vi "Calculate 1 digit.vi"(6 "index":i32, 7 "Digits":i32[](array[numeric])=[9, 8, 7, 6, 5, 4, 3, 2, 1], 9 "z out":i64, 10 "Input":string[](array[string])) -> (2 "Valid Inputs":cluster{i32, i32}[](array[cluster]))   [LabVIEW 2021]
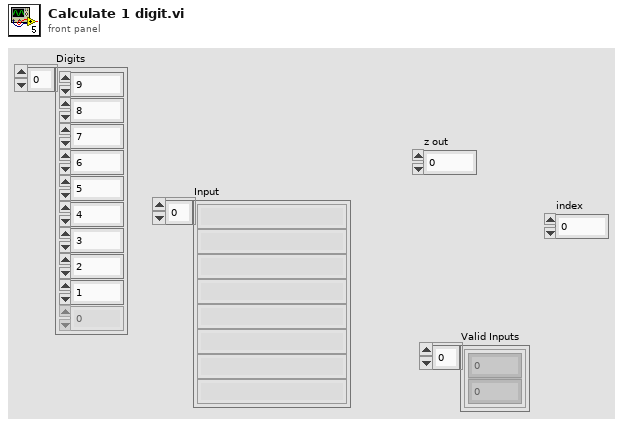
[diagram p1: front panel]
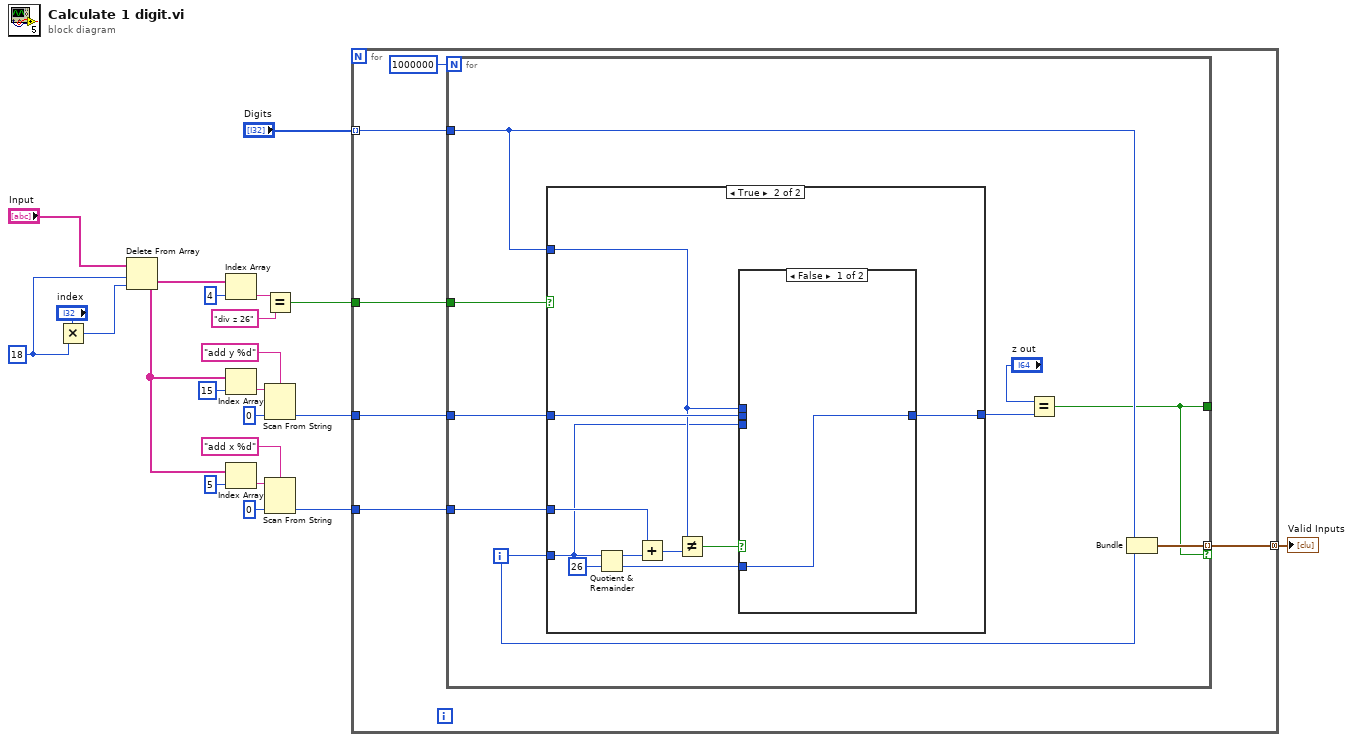
[diagram p0: block diagram]
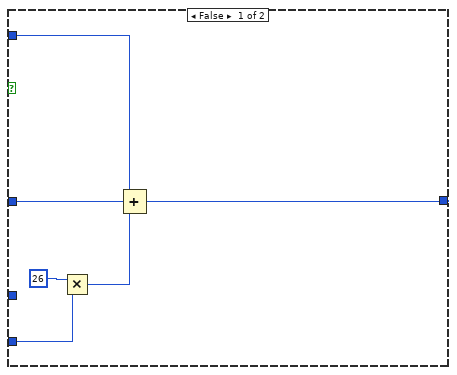
[diagram p2: hidden frame]
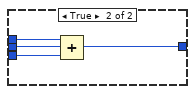
[diagram p3: hidden frame]
diagram:
  w5 = 18 ("length")
  n1 = Multiply(x="index", y=w5) -> (x*y=w3:i32)
  n2 = Delete From Array(array="Input", length=w5, index=w3) -> (deleted portion=w7:string[])  [unwired: 1 out]
  n3 = Index Array(array=w7, index=4) -> (element=w20:string)
  n4 = Index Array(array=w7, index=15) -> (element=w15:string)
  n5 = Index Array(array=w7, index=5) -> (element=w9:string)
  n6 = Equal?(x=w20, y="div z 26") -> (x = y?=w18:bool)
  n7 = Scan From String(format string="add y %d" ("y"), input string=w15, default 1=i64 0 ("default value 1")) -> (output 1=w12:i64)  [unwired: 2 in, 3 out]
  n8 = Scan From String(format string="add x %d" ("y"), input string=w9, default 1=i64 0 ("default value 1")) -> (output 1=w6:i64)  [unwired: 2 in, 3 out]
  n9 = for {
    tunnel: w18 -> [w27]
    tunnel: w12 -> [w26]
    tunnel: w6 -> [w25]
    tunnel: "Digits" -> [w24] mode=indexing
    tunnel: [w23] -> w2 mode=concatenating
    n10 = for {
      N: 1000000 -> [_]
      tunnel: w27 -> [w36]
      tunnel: w26 -> [w35]
      tunnel: w25 -> [w34]
      tunnel: w24 -> [w29]
      tunnel: [w28] -> _
      tunnel: [w30] -> w23 mode=indexing if=w28
      i -> [w31]
      n11 = case shown="True" w36 {
        tunnel: w29 -> [w40 w46]
        tunnel: w31 -> [w42 w43]
        tunnel: w35 -> [w38 w47]
        tunnel: [w37 w45] -> w32
        tunnel: w34 -> [_ w48]
        frame False {
          n12 = Multiply(x=i64 26 ("y"), y=w42) -> (x*y=w39:i64)
          n13 = Compound Arithmetic op=ADD(w40, w38, w39) -> (w37:i64)
        }
        frame True {
          n14 = Quotient & Remainder(x=w43, y=i64 26) -> (x-y*floor(x/y)=w51:i64, floor(x/y)=w44:i64)
          n15 = Add(x=w48, y=w51) -> (x+y=w50:i64)
          n16 = Not Equal?(x=w46, y=w50) -> (x != y?=w49:bool)
          n17 = case shown="False" w49 {
            tunnel: w47 -> [_ w57]
            tunnel: w46 -> [_ w56]
            tunnel: [w53 w55] -> w45
            tunnel: w44 -> [w53 _]
            tunnel: w43 -> [_ w54]
            frame False {
            }
            frame True {
              n18 = Compound Arithmetic op=ADD(w56, w57, w54) -> (w55:i64)
            }
          }
        }
      }
      n19 = Equal?(x="z out", y=w32) -> (x = y?=w28:bool)
      n20 = Bundle(w29, w31) -> (w30:cluster{i32, i32})  [unwired: 1 in]
    }
  }
  "Valid Inputs" <- w2
